vi "lvEtherbone.device_read_write.vi"(0 "eb_socket_ID":i32, 1 "eb_device_ID":i32, 2 "addressR":u64, 3 "timeout [ms]":i32=1000, 5 "error in (no error)":errorcluster, 6 "addressW":u64, 8 "modeW":T1 items=["EB_UNDEFINED"=-1, "EB_FIFO"=0, "EB_LINEAR"=1], 9 "modeR":T1 items=["EB_UNDEFINED"=-1, "EB_FIFO"=0, "EB_LINEAR"=1], 10 "dataW":u64[](array[numeric]), 11 "nR":i32) -> (13 "eb_status":T2, 14 "eb_socket_ID out":i32, 15 "eb_device_ID out":i32, 16 "dataR":u64[](array[numeric]), 17 "timed out?":bool, 19 "error out":errorcluster)   [LabVIEW 2009, in "lvEtherbone.lvlib"]
doc: "//-----------------------------------------------------------------------------------\n// author : Dietrich Beck, GSI-Darmstadt\n// purpose : Performs reading and writing to a Wishbone device\n// It is the responsibility of the caller to allocate memory for dataR (dataW)\n// The (preallocated) memory must have a size of 8*nR (8*nW) bytes. \n// returns : lveb_status_t\n//-----------------------------------------------------------------------------------\nETHERBONE_API int lveb_device_read_write( int eb_deviceID, //ID of Wishbone device\n uint64_t addressR, //address to read\n int modeR, //mode for reading (eb_mode_t)\n int nR, //number of read operations; no reading if 0\n uint64_t *dataR, //data that is read\n uint64_t addressW, //address to write\n int modeW, //mode for writing (eb_mode_t)\n int nW, //number of write operations; no writing if 0\n uint64_t *dataW, //data that is written\n int timeout //timeout [ms]\n );"
uses:
  lvEtherbone.lvlib
  lvEtherbone.lveb_status_t.ctl
  lvEtherbone.eb_mode_t.ctl
  bin/lvEtherbone.dll
panel:
  in  "myeb_status_t":T2
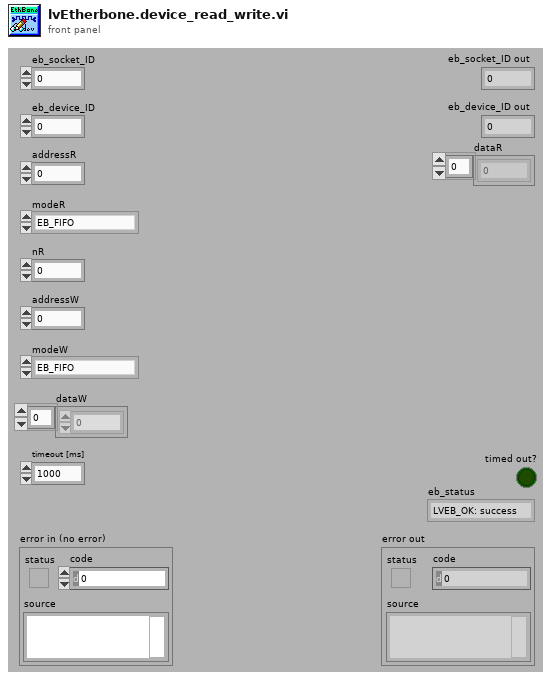
[diagram p1: front panel]
types:
  T1 = typedef "lvEtherbone.lvlib/lvEtherbone.eb_mode_t.ctl" = i32
  T2 = typedef "lvEtherbone.lvlib/lvEtherbone.lveb_status_t.ctl" = enum32{"LVEB_OK: success", "LVEB_UNKNOWN: unknown error", "LVEB_OS: operating system forbids access", "LVEB_PORT: port in use or unavailable", "LVEB_ID: ID invalid or out of resources", "LVEB_SOCKET: socket invalid or unavailable", "LVEB_EB: remote address is not Etherbone conformant", "LVEB_IP: bad format or network address", "LVEB_PORTWIDTH: port width error", "LVEB_DEVICEBUSY: Etherbone device still busy", "LVEB_DEVICEFAIL: operation on Wishbone device failed", "LVEB_DEVICEEXIST: Etherbone device already exists, overlaps, or does not exist", "LVEB_TIMEDOUT: a timeout occurred", "LVEB_OVERFLOW: payload of Etherbone exceeded", "LVEB_ADDRESS: bad address", "LVEB_ADDRESSWIDTH: address width error"}
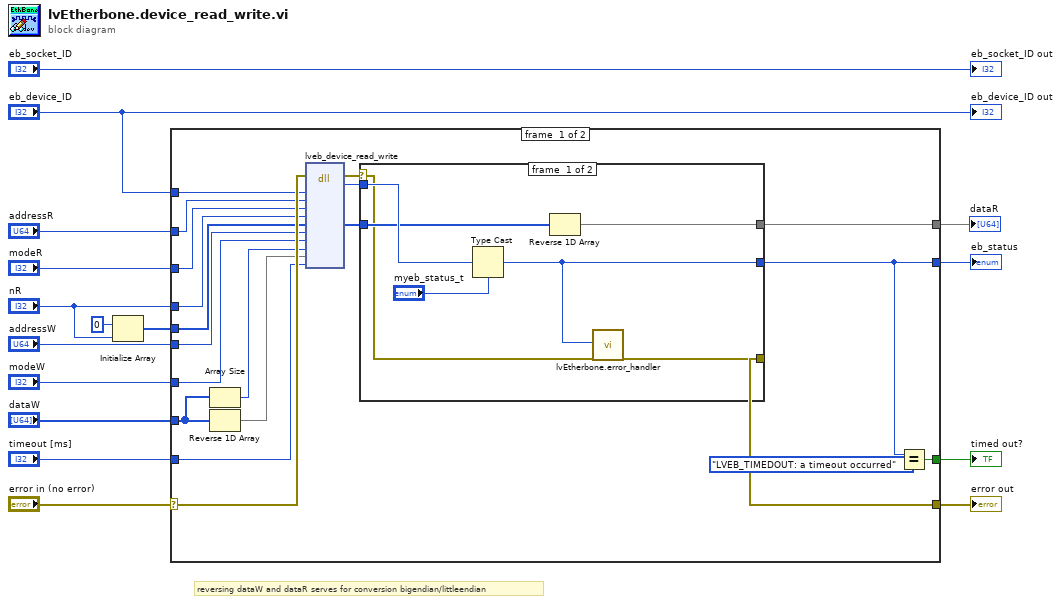
[diagram p0: block diagram]
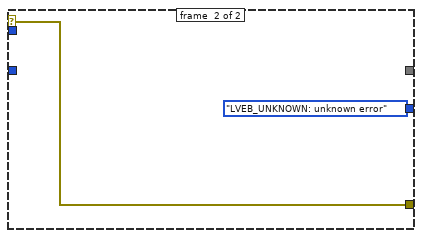
[diagram p2: hidden frame]
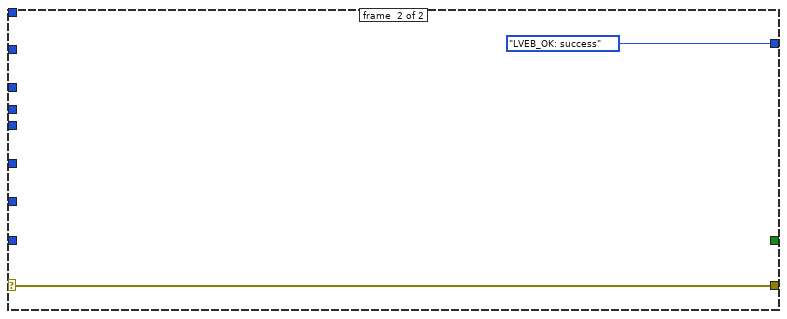
[diagram p3: hidden frame]
diagram:
  # "reversing dataW and dataR serves for conversion bigendian/littleendian"
  n1 = Initialize Array(u64 0 ("element"), "nR") -> (w1:u64[])
  n2 = case shown="No Error" "error in (no error)" {
    selector: "error in (no error)" -> [w36 w47]
    tunnel: [w31 w47] -> w15
    tunnel: "eb_device_ID" -> [w35 _]
    tunnel: "addressR" -> [w34 _]
    tunnel: "timeout [ms]" -> [w25 _]
    tunnel: [w29 lvEtherbone.lveb_status_t."LVEB_OK: success" ("eb_status_t")] -> w11
    tunnel: [w30 _] -> w4
    tunnel: [w27 _] -> w9
    tunnel: "modeR" -> [w26 _]
    tunnel: "nR" -> [w24 _]
    tunnel: "addressW" -> [w23 _]
    tunnel: "modeW" -> [w22 _]
    tunnel: "dataW" -> [w21 _]
    tunnel: w1 -> [w18 _]
    frame #0 {
      n3 = Array Size(array=w21) -> (size(s)=w20:i32)
      n4 = Reverse 1D Array(array=w21) -> (reversed array=w17:u64[])
      n5 = dll-call lib="F:/beck/Project/BEL/SCC/etherbone-core/api/lvEtherbone/bin/lvEtherbone.*" fn="lveb_device_read_write"(error in=w36, "eb_deviceID"=w35, "addressR"=w34, "modeR"=w26, "nR"=w24, "dataR"=w18, "addressW"=w23, "modeW"=w22, "nW"=w20, "dataW"=w17, "timeout"=w25) -> (error out=w33:errorcluster, "myeb_status"=w32:i32, "dataR"=w19:u64[])  [unwired: 11 in, 1 out]
      n6 = case shown="No Error" w33 {
        selector: w33 -> [w38 w45]
        tunnel: w32 -> [w43 _]
        tunnel: [w40 lvEtherbone.lveb_status_t."LVEB_UNKNOWN: unknown error" ("eb_status_t")] -> w29
        tunnel: [w39 w45] -> w31
        tunnel: w19 -> [w42 _]
        tunnel: [w37 _] -> w30
        frame #0 {
          n7 = Type Cast(type="myeb_status_t", x=w43) -> (*(type *) &x=w40:T2)
          n8 = Reverse 1D Array(array=w42) -> (reversed array=w37:u64[])
          n9 = call "lvEtherbone.error_handler.vi"("eb_status"=w40, "error in"=w38) -> ("error out"=w39:errorcluster)  [unwired: 17 in]
        }
        frame #1 {
        }
      }
      n10 = Equal?(x=w29, y=lvEtherbone.lveb_status_t."LVEB_TIMEDOUT: a timeout occurred") -> (x = y?=w27:bool)
    }
    frame #1 {
    }
  }
  "error out" <- w15
  "eb_status" <- w11
  "timed out?" <- w9
  "dataR" <- w4
  "eb_socket_ID out" <- "eb_socket_ID"
  "eb_device_ID out" <- "eb_device_ID"
